vi "HTTP_GET_Test_RemoveOneUserData.vi"(8 "error in (no error)":errorcluster, 11 "ReqNum":string) -> (0 "error out":errorcluster, 3 "body 2":string)   [LabVIEW 2017]
uses:
  <vilib>/httpClient/LabVIEWHTTPClient.lvlib
panel:
  out "headers 2":string
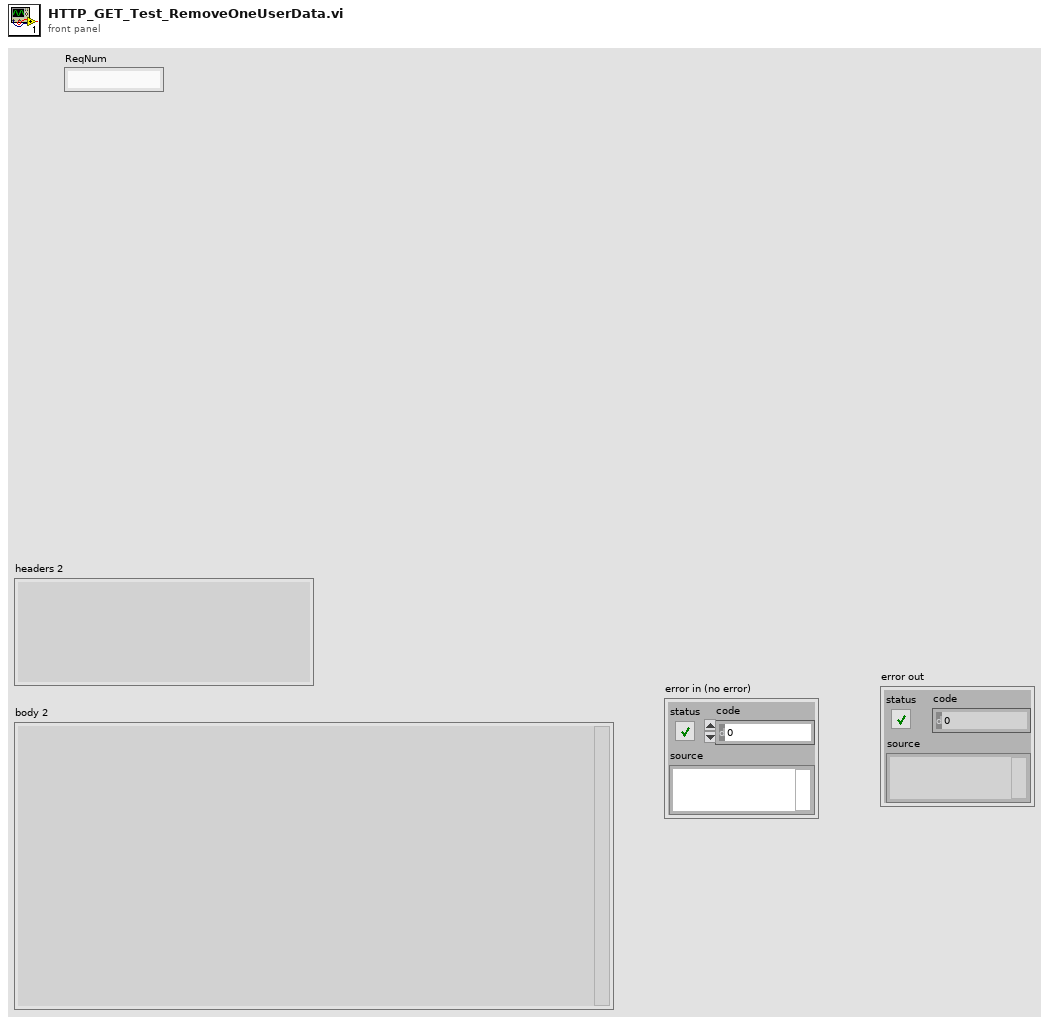
[diagram p1: front panel]
types:
  T1 = typedef "LabVIEWHTTPClient.lvlib/ClientHandle.ctl" = refnum<k1>
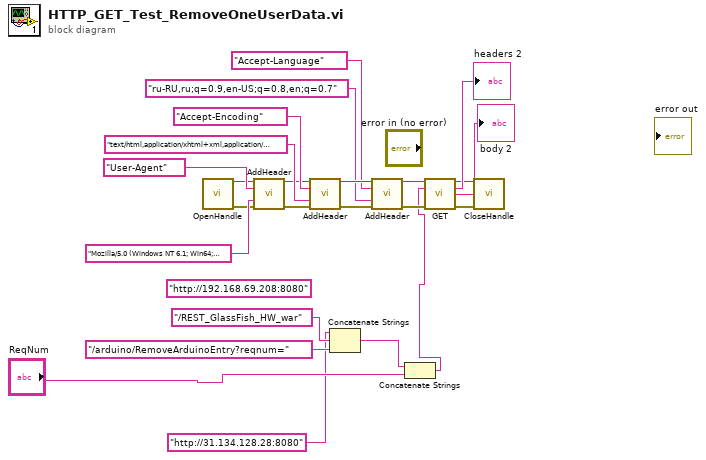
[diagram p0: block diagram]
diagram:
  (unwired) "http://192.168.69.208:8080" ("url")
  n1 = call <vilib>:"OpenHandle.vi"() -> ("client handle out"=w7:T1, "error out"=w8:errorcluster)  [unwired: 14 in]
  n2 = call <vilib>:"AddHeader.vi"("client handle"=w7, "header"="User-Agent", "value"="Mozilla/5.0 (Windows NT 6.1; Win64; x64) AppleWebKit/537.36 (KHTML, like Gecko) Chrome/75.0.3770.100 Safari/537.36", "error in (no error)"=w8) -> ("client handle out"=w11:T1, "error out"=w12:errorcluster)  [unwired: 10 in]
  n3 = call <vilib>:"AddHeader.vi"("client handle"=w11, "header"="Accept-Encoding", "value"="text/html,application/xhtml+xml,application/xml;q=0.9,image/webp,image/apng,*/*;q=0.8,application/signed-exchange;v=b3", "error in (no error)"=w12) -> ("client handle out"=w17:T1, "error out"=w18:errorcluster)  [unwired: 10 in]
  n4 = Concatenate Strings("http://31.134.128.28:8080" ("url"), "/REST_GlassFish_HW_war" ("url"), "/arduino/RemoveArduinoEntry?reqnum=" ("url")) -> (w4:string)
  n5 = call <vilib>:"AddHeader.vi"("client handle"=w17, "header"="Accept-Language", "value"="ru-RU,ru;q=0.9,en-US;q=0.8,en;q=0.7", "error in (no error)"=w18) -> ("client handle out"=w19:T1, "error out"=w20:errorcluster)  [unwired: 10 in]
  n6 = Concatenate Strings(w4, "ReqNum") -> (w3:string)
  n7 = call <vilib>:"GET.vi"("client handle"=w19, "url"=w3, "error in (no error)"=w20) -> ("client handle out"=w21:T1, "headers"=→"headers 2":string, "body"=→"body 2":string, "error out"=w22:errorcluster)  [unwired: 9 in]
  n8 = call <vilib>:"CloseHandle.vi"("client handle"=w21, "error in (no error)"=w22) -> ()  [unwired: 13 in, 1 out]
